vi "filter_test.vi"() -> ()   [LabVIEW 2013]
uses:
  <vilib>/rvi/FXPMathLib/FxpConvert/subVIs/nifxpmath_Convert_SimConfig.ctl
  <vilib>/fxp/LVFixedPointQuantizationPolicyTypeDef.ctl
  <vilib>/fxp/LVFixedPointOverflowPolicyTypeDef.ctl
  <vilib>/rvi/FXPMathLib/FxpConvert/simVIs/DllFxpConvertTemp_sub.vi
  <vilib>/rvi/FXPMathLib/FxpInterpret/XNode/nifxpmath_Interpret.xnode
  <vilib>/rvi/FXPMathLib/FxpConvert/XNode/nifxpmath_Convert.xnode
panel:
  out "size(s)":i32
  out "logical OR":bool
  out "Array 2":bool[](array[boolean])
  out "Array":fxp<+/-,16,16>[](array[numeric])
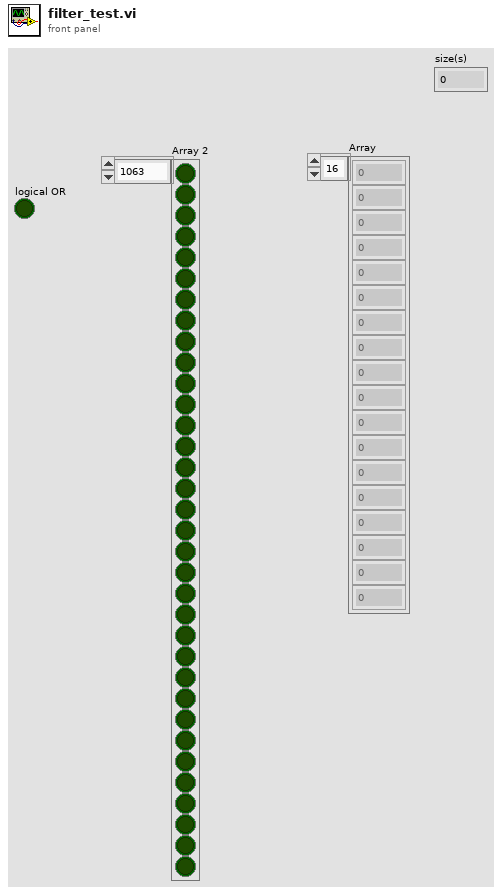
[diagram p1: front panel]
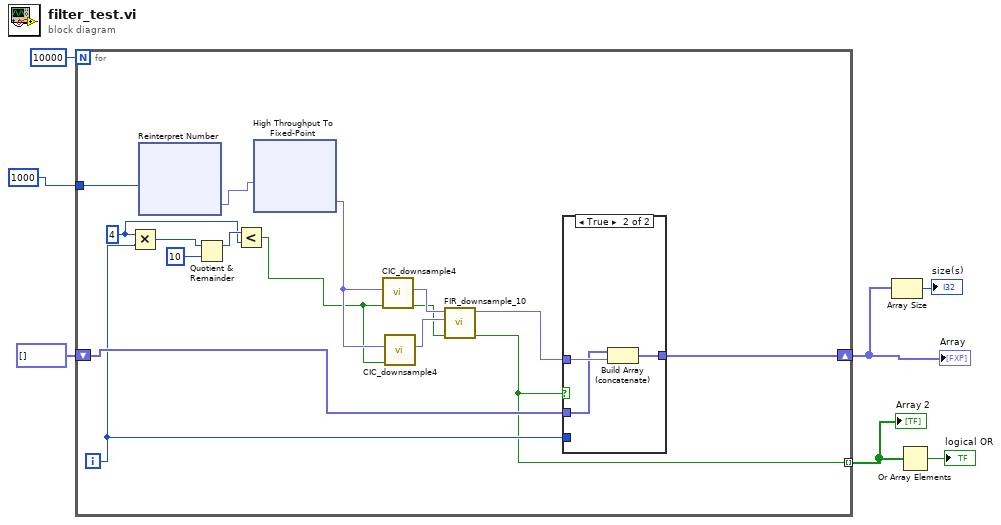
[diagram p0: block diagram]
diagram:
  n1 = for {
    N: 10000 -> [_]
    shift-right: [w21] -> w3
    shift-left: fxp<+/-,16,16>[] [] -> [w20]
    tunnel: [w8] -> w4 mode=indexing
    tunnel: 1000 -> [w15]
    i -> [w14]
    w11 = 4 ("x")
    n2 = Multiply(x=w11, y=w14) -> (x*y=w13:i32)
    n3 = xnode "Reinterpret Number"("x"=w15) -> ("y"=w22:fxp<+/-,32,32>)
    n4 = Quotient & Remainder(x=w13, y=10) -> (x-y*floor(x/y)=w12:i32)  [unwired: 1 out]
    n5 = Less?(x=w12, y=w11) -> (x < y?=w10:bool)
    n6 = xnode "High Throughput To Fixed-Point"("x"=w22) -> ("y"=w18:fxp<+/-,20,16>)
    n7 = call "CIC_downsample4.vi"("valid in"=w10, "din"=w18) -> ("valid out"=w9:bool, "dout"=w19:fxp<+/-,25,19>)  [unwired: 7 in, 1 out]
    n8 = call "CIC_downsample4.vi"("valid in"=w10, "din"=w18) -> ("dout"=w17:fxp<+/-,25,19>)  [unwired: 7 in, 2 out]
    n9 = call "FIR_downsample_10.vi"("valid in"=w9, "Q in"=w17, "I in"=w19) -> ("valid out"=w8:bool, "I out"=w16:fxp<+/-,16,16>)  [unwired: 6 in, 1 out]
    n10 = case shown="True" w8 {
      tunnel: w16 -> [_ w27]
      tunnel: [w24 w26] -> w21
      tunnel: w20 -> [w24 w25]
      tunnel: w14 -> [_ _]
      frame False {
      }
      frame True {
        n11 = Build Array (concatenate)(w25, w27) -> (w26:fxp<+/-,16,16>[])
      }
    }
  }
  "Array" <- w3
  "Array 2" <- w4
  n12 = Array Size(array=w3) -> (size(s)=→"size(s)":i32)
  n13 = Or Array Elements(Boolean array=w4) -> (logical OR=→"logical OR":bool)
